vi "FTW-Test-ActorInitFailed.vi"() -> (0 "error out":errorcluster)   [LabVIEW 2015]
uses:
  Test Actor/core/FTW-Test-Actor-Core_Process.vi
  source/actor/Connector/FTW-ActorConnector.lvclass
  source/actor/Ether/FTW-Ether.lvclass
  Test Actor/core/FTW-Test-Actor-Core.lvclass
panel:
  out "Response Body":string
  out "Instance Inbox Address":string
  out "Initialized Response":string
  out "Timed out?":bool
  out "Ping Response":string
  in  "FTW Ether Configuration":string="{\n  \"ApplicationName\": \"Actor Example\",\n  \"ApplicationVersion\": \"0.1.0-1\",\n  \"LoggerAddress\": \"inproc://*\",\n  \"LoggerName\": \"ActorExample\",\n  \"LoggerDirectory\": \"[UserDesktop]\\\\Logs\",\n  \"LoggerDiskThrashDelay\": 200\n}"
  in  "Actor 1 Configuration":string="{\n  \"Identity\": \"Test Actor\",\n  \"InboxAddress\": \"inproc://*\",\n  \"LoggerAddress\": \"\",\n  \"Fail Initialization\": true\n}"
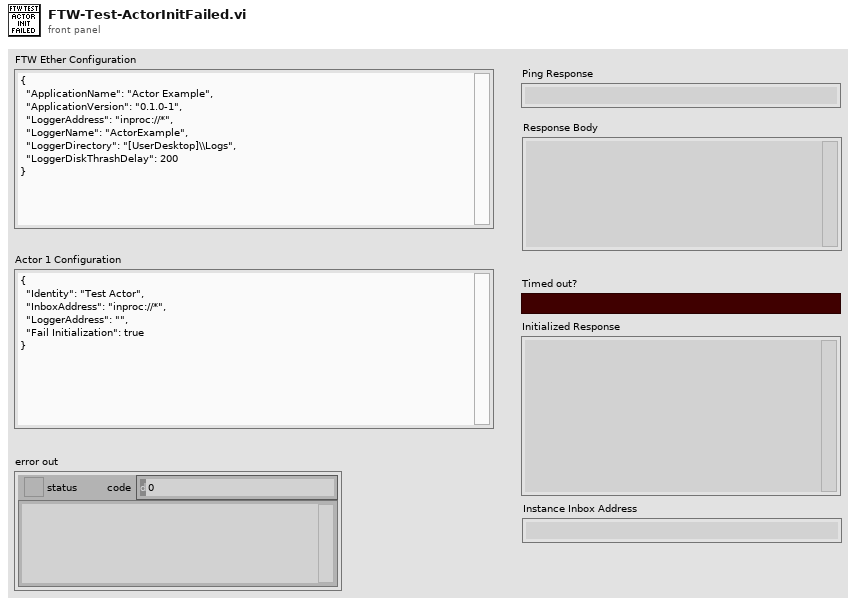
[diagram p1: front panel]
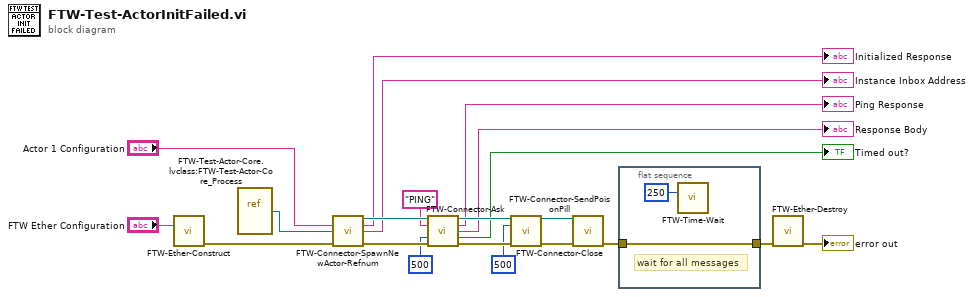
[diagram p0: block diagram]
diagram:
  n1 = call "FTW-Ether-Construct.vi"("FTW Ether Configuration"="FTW Ether Configuration") -> ("error out"=w18:errorcluster)  [unwired: 14 in]
  n2 = vi-ref "FTW-Test-Actor-Core.lvclass:FTW-Test-Actor-Core_Process.vi"() -> (w2:refnum<vi>)
  n3 = call "FTW-Connector-SpawnNewActor-Refnum.vi"("Configuration"="Actor 1 Configuration", "Actor VI Refnum"=w2, "error in"=w18) -> ("FTW Actor Connector"=w21:refnum<class "FTW-ActorConnector.lvclass">, "Initialized Response"=→"Initialized Response":string, "Instance Inbox Address"=→"Instance Inbox Address":string, "error out"=w10:errorcluster)  [unwired: 9 in]
  n4 = call "FTW-Connector-Ask.vi"("FTW Actor Connector"=w21, "Request Header"="PING", "Timeout"=500, "error in"=w10) -> ("FTW Actor Connector out"=w20:refnum<class "FTW-ActorConnector.lvclass">, "Response Header"=→"Ping Response":string, "Response Body"=→"Response Body":string, "Timed out?"=→"Timed out?":bool, "error out"=w8:errorcluster)  [unwired: 6 in, 1 out]
  n5 = call-dynamic "FTW-Connector-SendPoisonPill.vi"("FTW Actor Connector"=w20, "Timeout"=500, "error in"=w8) -> ("FTW Actor Connector out"=w7:refnum<class "FTW-ActorConnector.lvclass">, "error out"=w6:errorcluster)  [unwired: 7 in, 4 out]
  n6 = call-dynamic "FTW-Connector-Close.vi"("FTW Actor Connector"=w7, "error in"=w6) -> ("error out"=w14:errorcluster)  [unwired: 13 in]
  n7 = flat-sequence {
    tunnel: w14 -> [w22]
    tunnel: [w22] -> w1
    frame #0 {
      # "wait for all messages"
      n8 = call "FTW-Time-Wait.vi"("Wait Time (ms)"=u32 250) -> ()  [unwired: 14 in, 1 out]
    }
  }
  n9 = call "FTW-Ether-Destroy.vi"("error in"=w1) -> ("error out"=→"error out":errorcluster)  [unwired: 14 in]
